vi "Read Gas.vi"(8 "error in":errorcluster, 11 "Alicat in":refnum<class "Alicat.lvclass">) -> (0 "error out":errorcluster, 2 "Gas":T1, 3 "Alicat out":refnum<class "Alicat.lvclass">)   [LabVIEW 2014, in "Alicat.lvlib" / "Alicat.lvclass"]
uses:
  Alicat.lvclass
  Controls/Gas.ctl
  Alicat.lvclass/Alicat.ctl
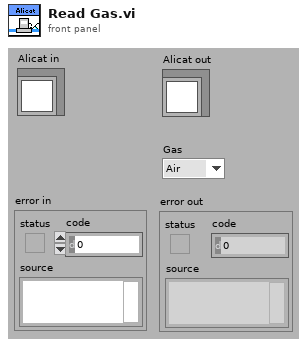
[diagram p1: front panel]
types:
  T1 = typedef "Alicat.lvlib/Alicat.lvclass/Gas.ctl" = enum16{"Air", "Ar", "CH4", "CO", "CO2", "C2H6", "H2", "He", "N2", "NO", "Ne", "O2", "C3H8", "n-C4H10", "C2H2", "C2H4", "i-C2H10", "Kr", "Xe"}
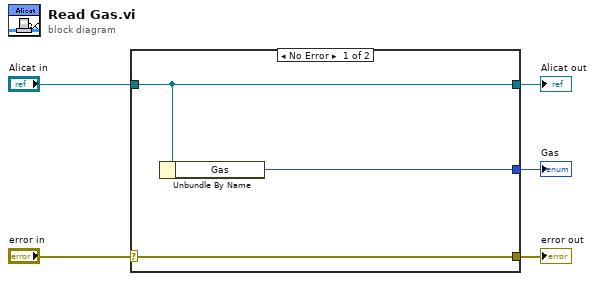
[diagram p0: block diagram]
diagram:
  n1 = case shown="No Error" "error in" {
    selector: "error in" -> [w8 w9]
    tunnel: [w8 w9] -> w4
    tunnel: [w7 w10] -> w2
    tunnel: "Alicat in" -> [w7 w10]
    tunnel: [w6 _] -> w1
    frame No Error {
      n2 = Unbundle By Name(w7) -> ("Gas"=w6:T1)
    }
    frame Error {
    }
  }
  "error out" <- w4
  "Alicat out" <- w2
  "Gas" <- w1
